vi "appendElement.vi"(7 "Document in":refnum<class "xwpfDocument.lvclass">, 8 "error in (no error)":errorcluster, 11 "xwpfTable in":refnum<class "xwpfTable.lvclass">) -> (0 "error out":errorcluster, 3 "xwpfTable out":refnum<class "xwpfTable.lvclass">, 5 "Document out":refnum<class "xwpfDocument.lvclass">)   [LabVIEW 2017, in "Word_Specific.lvlib" / "xwpfTable.lvclass"]
uses:
  xwpfTable.lvclass
  xwpfDocument/xwpfDocument.lvclass
  xwpfTable.lvclass/xwpfTable.ctl
  xwpfParagraph/xwpfParagraph.lvclass/xwpfParagraph.ctl
  xwpfRun/xwpfRun.lvclass/xwpfRun.ctl
  xwpfRun/Get Text.vi
  xwpfRun/Get Style.vi
  xwpfParagraph/Get Runs.vi
  Get Cells.vi
  xwpfParagraph/xwpfParagraph.lvclass
  xwpfRun/xwpfRun.lvclass
  Styles/Style/Style.lvclass
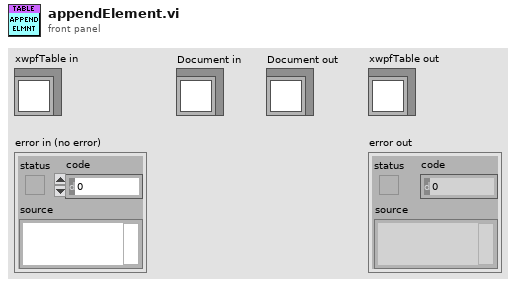
[diagram p1: front panel]
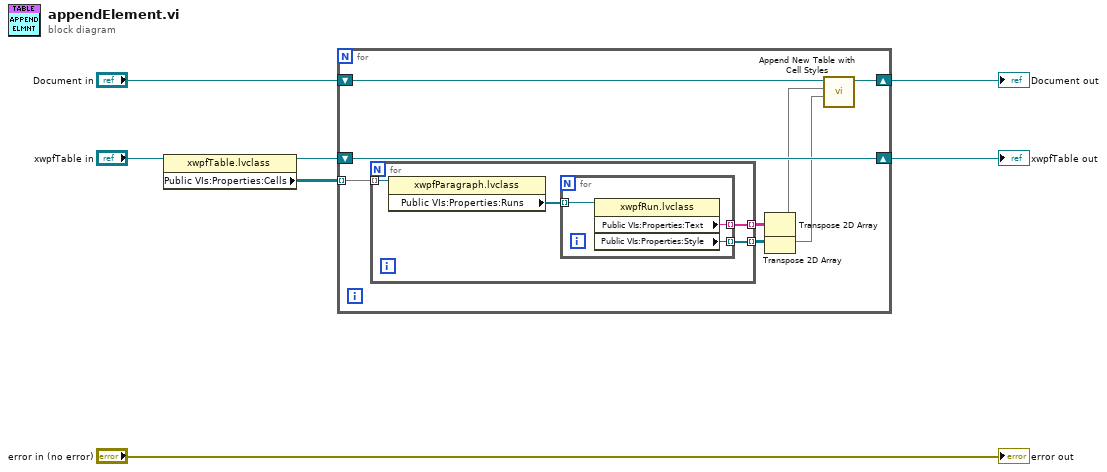
[diagram p0: block diagram]
diagram:
  n1 = property class="xwpfTable.lvclass"(reference="xwpfTable in") -> (reference out=w4:refnum<class "xwpfTable.lvclass">, "Public VIs:Properties:Cells"=w5:refnum<class "xwpfParagraph.lvclass">[][])  [unwired: 1 in, 1 out]
  n2 = for {
    tunnel: w5 -> [w12] mode=indexing
    shift-right: [w15] -> w3
    shift-left: w4 -> [w15]
    shift-right: [w13] -> w1
    shift-left: "Document in" -> [w14]
    n3 = for {
      tunnel: w12 -> [w19] mode=indexing
      tunnel: [w17] -> w11 mode=indexing
      tunnel: [w16] -> w9 mode=indexing
      n4 = property class="xwpfParagraph.lvclass"(reference=w19) -> ("Public VIs:Properties:Runs"=w18:refnum<class "xwpfRun.lvclass">[])  [unwired: 1 in, 2 out]
      n5 = for {
        tunnel: w18 -> [w22] mode=indexing
        tunnel: [w21] -> w17 mode=indexing
        tunnel: [w20] -> w16 mode=indexing
        n6 = property class="xwpfRun.lvclass"(reference=w22) -> ("Public VIs:Properties:Text"=w21:string, "Public VIs:Properties:Style"=w20:refnum<class "Style.lvclass">)  [unwired: 1 in, 2 out]
      }
    }
    n7 = Transpose 2D Array(2D array=w11) -> (transposed array=w10:string[][])
    n8 = Transpose 2D Array(2D array=w9) -> (transposed array=w8:refnum<class "Style.lvclass">[][])
    n9 = call "Append New Table with Cell Styles.vi"("Cell.Styles"=w8, "Table.Data"=w10, "xwpfDocument in"=w14) -> ("xwpfDocument out"=w13:refnum<class "xwpfDocument.lvclass">)  [unwired: 7 in, 1 out]
  }
  "xwpfTable out" <- w3
  "Document out" <- w1
  "error out" <- "error in (no error)"
